vi "ScanParams.vi"(0 "Probe":T2(ring)=enum."Hit U533 Ang6 Sag", 1 "Multiframes?":bool, 7 "hide ftp option? in":bool=TRUE, 9 "location in":u16(ring)=3 items=["VMMC", "U_HI", "Sloan Kett", "Columbia", "RRI Test"], 11 "GaGe Mem":dbl=3.0) -> (4 "Machine Params":T1 {"Scan Info"."sector scan angle" format="%.2f"; "Scan Info"."pivot distance" format="%.2f"; "Scan Info"."delay" format="%.2f"}, 6 "Distance between\nscan lines (um)":sgl, 8 "directory to save data out":path, 10 "hide ftp option? out":bool, 13 "FTP params":T3, 15 "location out":u16(ring)=3 items=["VMMC", "U_HI", "Sloan Kett", "Columbia", "RRI Test"])   [LabVIEW 2022 SP3]
uses:
  MachineParams.ctl
panel:
  out "trig depth pts":dbl
  in  "directory to save data in":path=path "D:/"
  # "Have to set ConterConfig.vi triggers for each machine type."
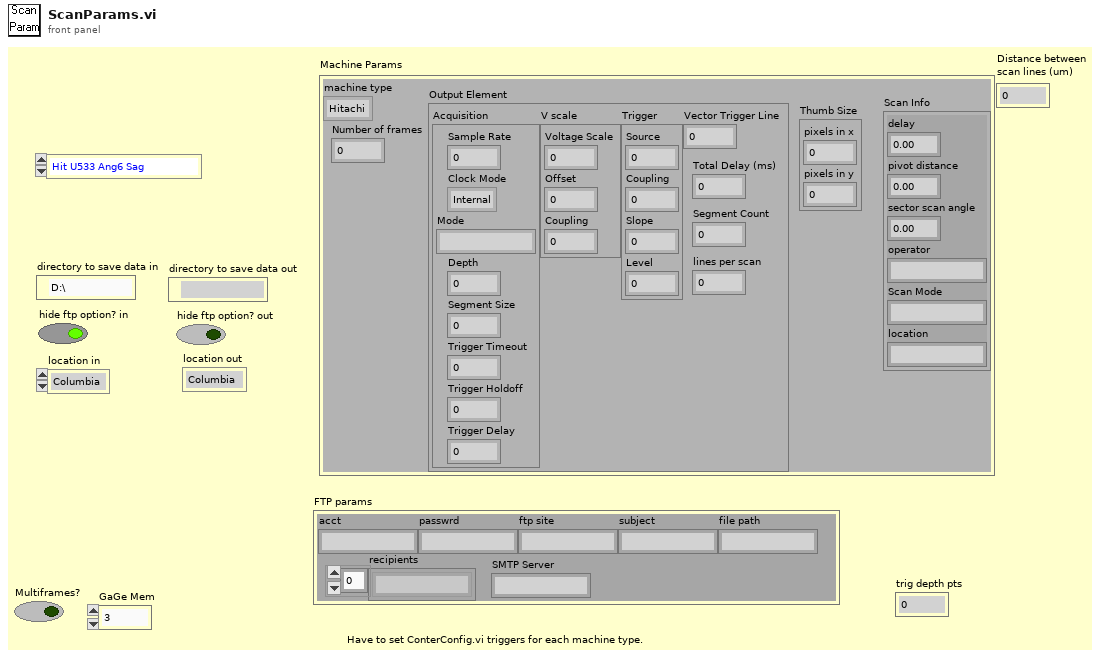
[diagram p1: front panel]
types:
  T1 = typedef "MachineParams.ctl" = cluster{"machine type":enum16{"Hitachi", "B&K 3535", "B&K Hawk"}, "Number of frames":dbl, "Output Element":cluster{"Acquisition":cluster{"Sample Rate":dbl, "Clock Mode":enum16{"Internal", "External", "Reference"}, "Mode":string, "Depth":dbl, "Segment Size":dbl, "Trigger Timeout":dbl, "Trigger Holdoff":dbl, "Trigger Delay":dbl}, "V scale":cluster{"Voltage Scale":i16, "Offset":dbl, "Coupling":u16}, "Trigger":cluster{"Source":u16, "Coupling":u16, "Slope":u16, "Level":dbl}, "Vector Trigger Line":i16, "Total Delay (ms)":dbl, "Segment Count":u32, "lines per scan":i32}, "Thumb Size":cluster{"pixels in x":i16, "pixels in y":i16}, "Scan Info":cluster{"delay":sgl, "pivot distance":sgl, "sector scan angle":sgl, "operator":string, "Scan Mode":string, "location":string}}
  T2 = enum16{"Hitachi-fast (Vx3W)", "Hitachi-detailed (Vx3W)", "Hit U533 Ang5 Trans", "Hit U533 Ang4 Trans", "Hit U533 Ang3 Trans", "Hit U533 Ang6 Sag", "B&K 3535 with TGC", "B&K 3535 with no TGC", "B&K Hawk 8808 (S)", "B&K Hawk 8808 (T)", "B&K Hawk 8808 (Split)", "B&K Hawk 8658 (S)", "B&K Hawk 8658 (T)", "B&K Hawk 8663"}
  T3 = cluster{"acct":string, "passwrd":string, "ftp site":string, "subject":string, "file path":string, "recipients":string[], "SMTP Server":string}
  T4 = cluster{"Acquisition":cluster{"Sample Rate":dbl, "Clock Mode":enum16{"Internal", "External", "Reference"}, "Mode":string, "Depth":dbl, "Segment Size":dbl, "Trigger Timeout":dbl, "Trigger Holdoff":dbl, "Trigger Delay":dbl}, "V scale":cluster{"Voltage Scale":i16, "Offset":dbl, "Coupling":u16}, "Trigger":cluster{"Source":u16, "Coupling":u16, "Slope":u16, "Level":dbl}, "Vector Trigger Line":i16, "Total Delay (ms)":dbl, "Segment Count":u32, "lines per scan":i32}
  T5 = cluster{"delay":sgl, "pivot distance":sgl, "sector scan angle":sgl, "operator":string, "Scan Mode":string, "location":string}
  T6 = cluster{string, string, string, string, string, "recipients":string[], string}
  T7 = cluster{enum16{"Hitachi", "B&K 3535", "B&K Hawk"}, dbl, "Output Element":cluster{"Acquisition":cluster{"Sample Rate":dbl, "Clock Mode":enum16{"Internal", "External", "Reference"}, "Mode":string, "Depth":dbl, "Segment Size":dbl, "Trigger Timeout":dbl, "Trigger Holdoff":dbl, "Trigger Delay":dbl}, "V scale":cluster{"Voltage Scale":i16, "Offset":dbl, "Coupling":u16}, "Trigger":cluster{"Source":u16, "Coupling":u16, "Slope":u16, "Level":dbl}, "Vector Trigger Line":i16, "Total Delay (ms)":dbl, "Segment Count":u32, "lines per scan":i32}, "Thumb Size":cluster{"pixels in x":i16, "pixels in y":i16}, "Scan Info":cluster{"delay":sgl, "pivot distance":sgl, "sector scan angle":sgl, "operator":string, "Scan Mode":string, "location":string}}
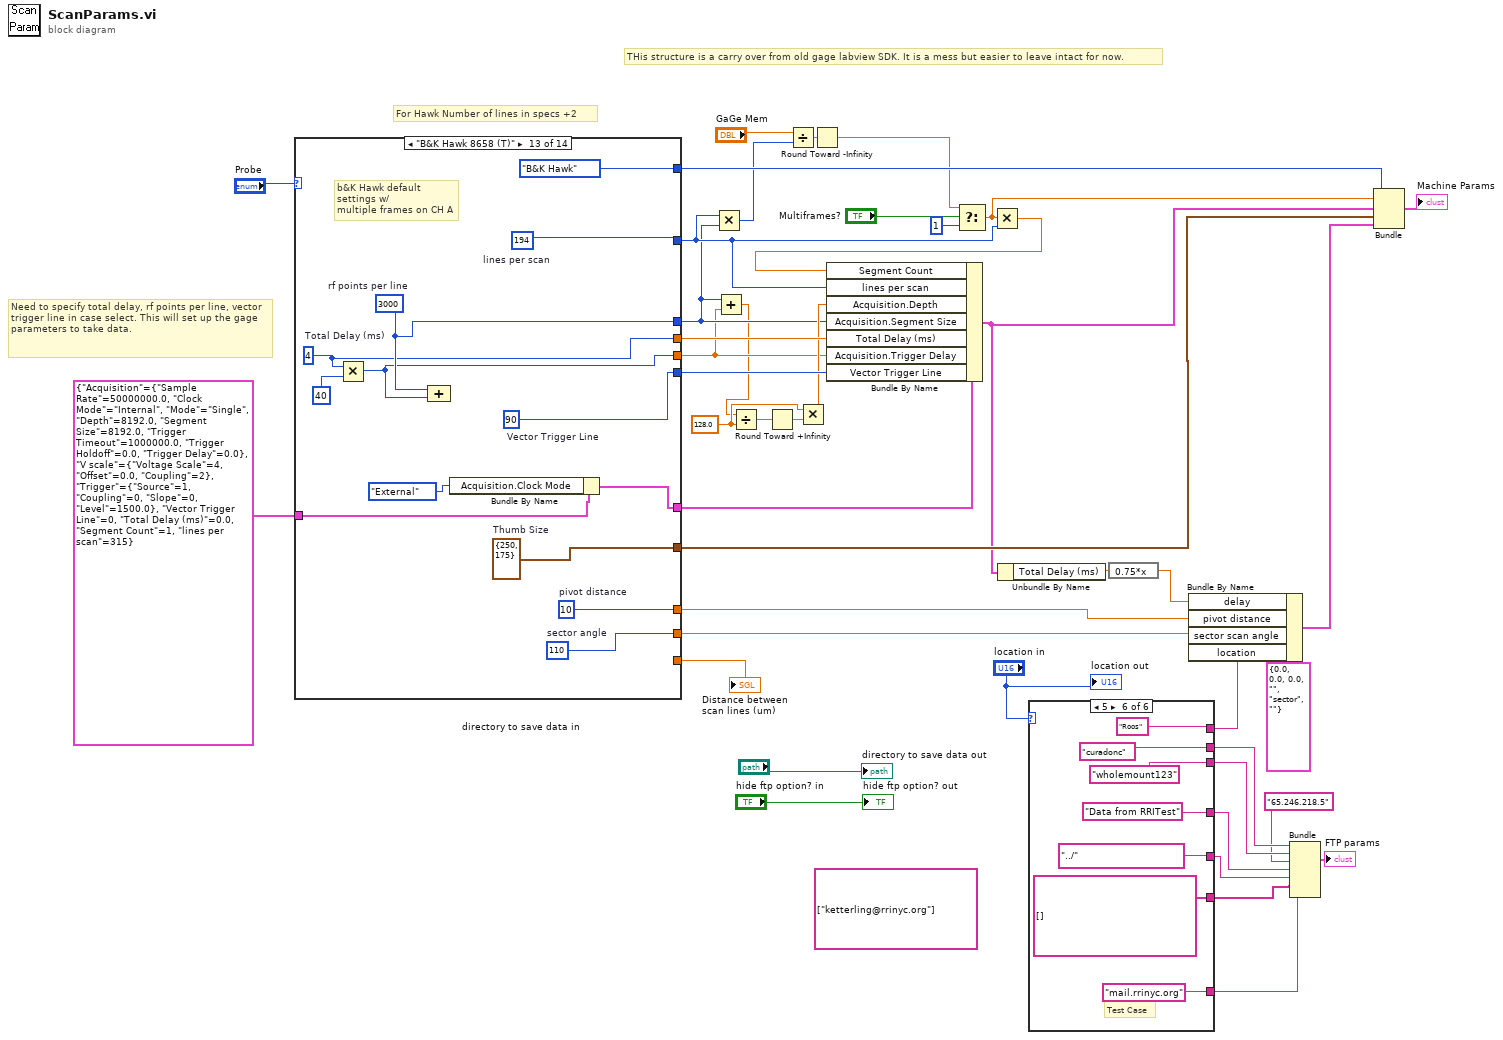
[diagram p0: block diagram]
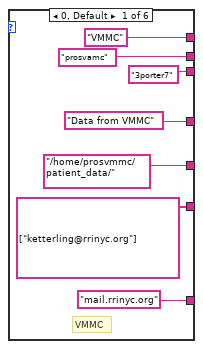
[diagram p2: hidden frame]
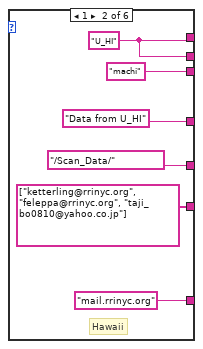
[diagram p3: hidden frame]
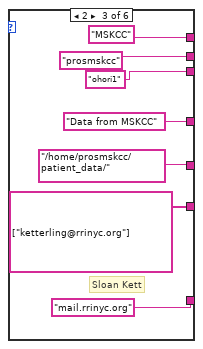
[diagram p4: hidden frame]
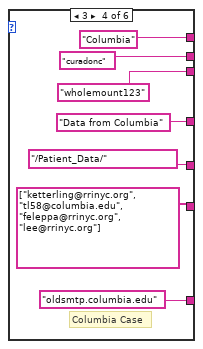
[diagram p5: hidden frame]
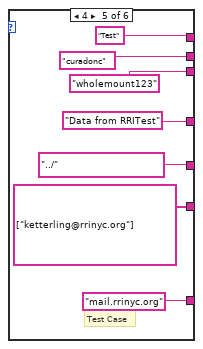
[diagram p6: hidden frame]
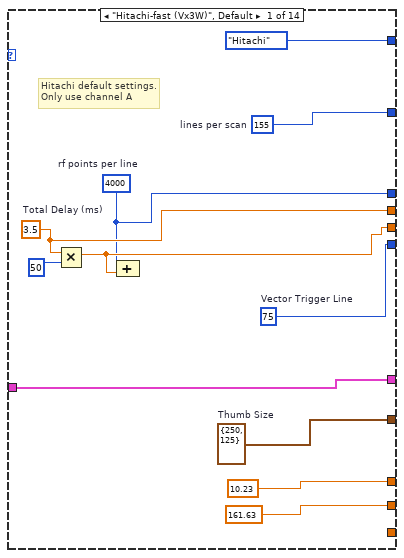
[diagram p7: hidden frame]
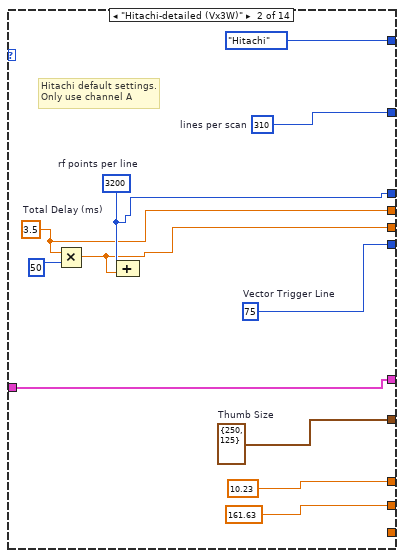
[diagram p8: hidden frame]
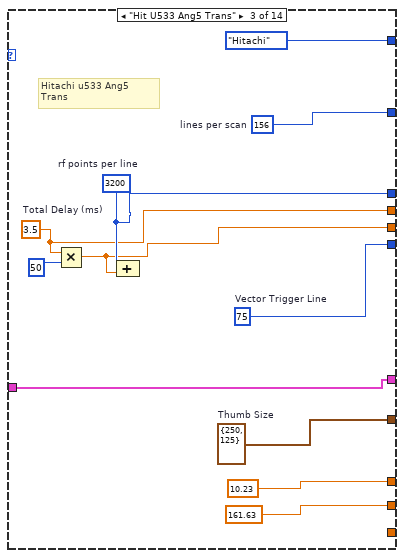
[diagram p9: hidden frame]
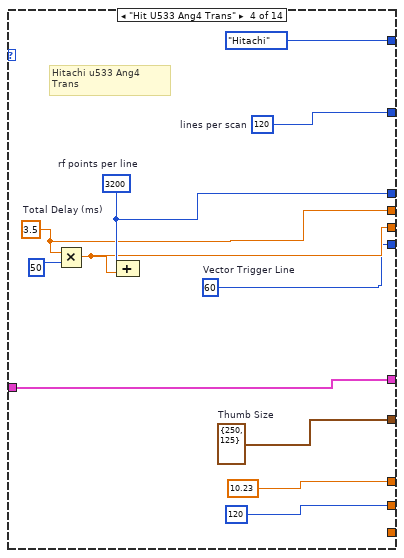
[diagram p10: hidden frame]
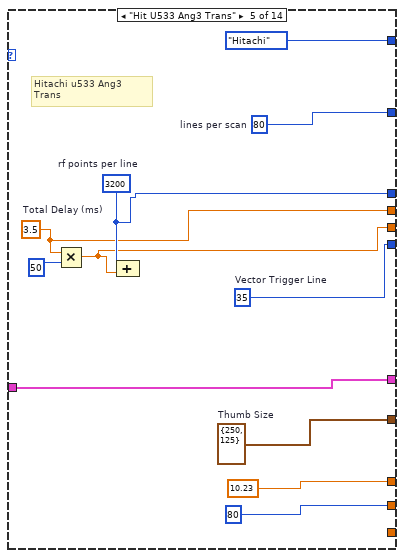
[diagram p11: hidden frame]
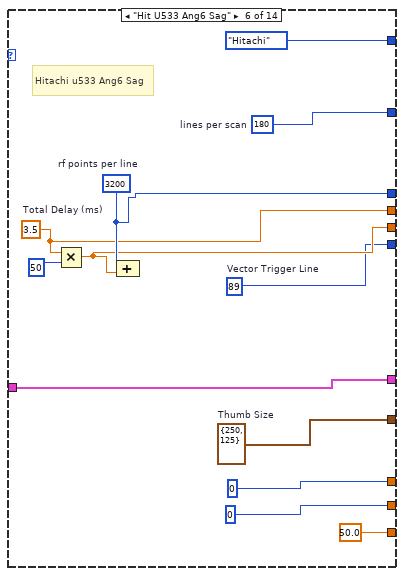
[diagram p12: hidden frame]
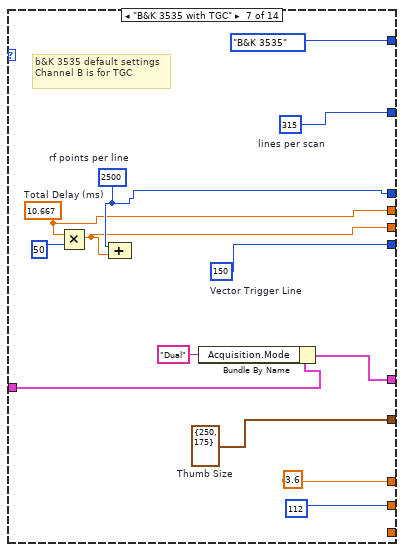
[diagram p13: hidden frame]
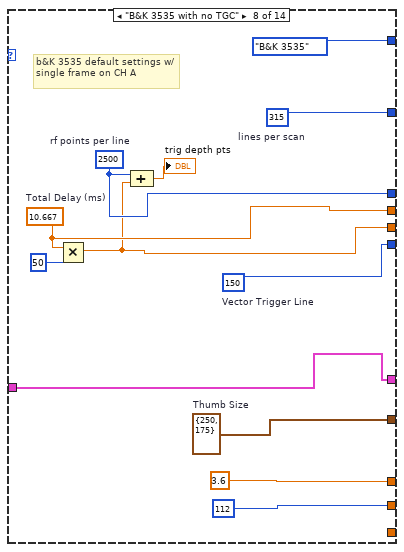
[diagram p14: hidden frame]
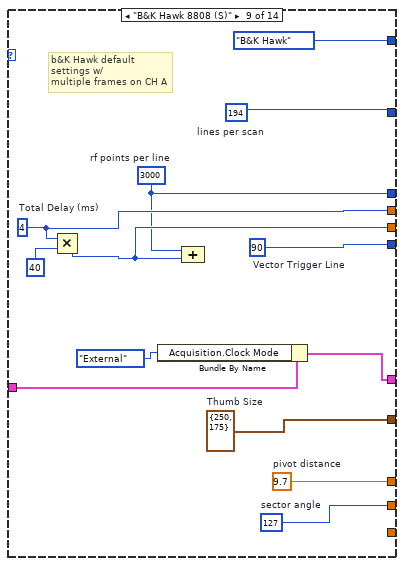
[diagram p15: hidden frame]
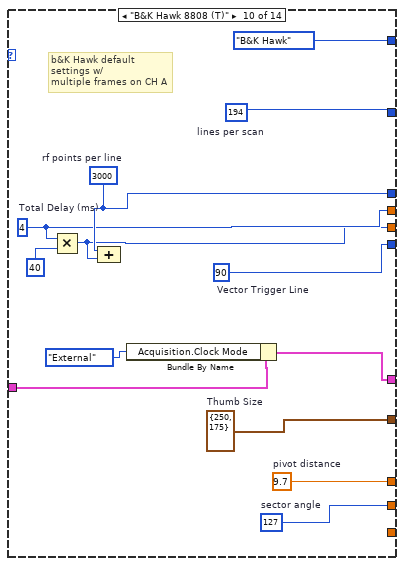
[diagram p16: hidden frame]
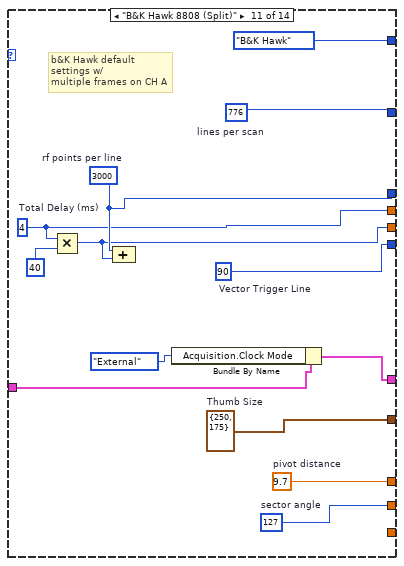
[diagram p17: hidden frame]
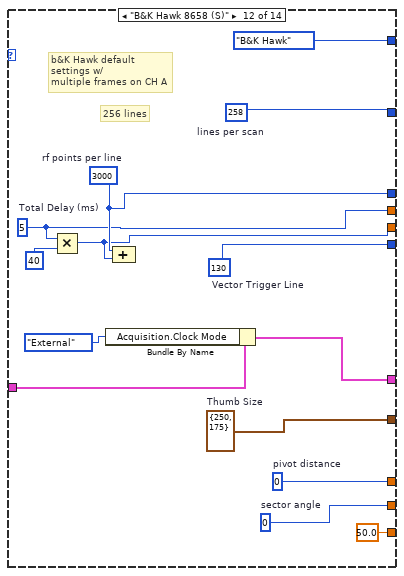
[diagram p18: hidden frame]
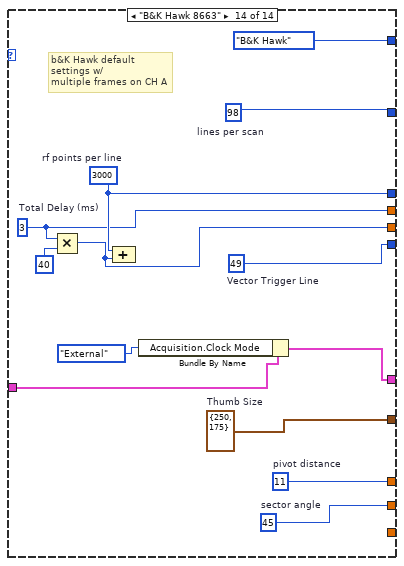
[diagram p19: hidden frame]
diagram:
  w8 = 128.0 ("y")
  (unwired) string[] ["ketterling@rrinyc.org"] ("recipients")
  # "THis structure is a carry over from old gage labview SDK. It is a mess but easier to leave intact for now."
  # "For Hawk Number of lines in specs +2"
  # "Need to specify total delay, rf points per line, vector trigger line in case select. This will set up the gage parameters to take data."
  n1 = case shown="\"B&K Hawk 8658 (T)\"" "Probe" {
    tunnel: [w50 w61 w72 w83 w94 w106 w119 w131 w144 w158 w171 w185 w198 w211] -> w14
    tunnel: [w55 w66 w77 w88 w99 w111 w124 w136 w149 w162 w175 w189 w202 w215] -> w20
    tunnel: [10.23 10.23 10.23 10.23 10.23 0 3.6 3.6 w148 w161 w174 w188 w201 w214] -> w41
    tunnel: [161.63 161.63 161.63 120 80 0 112 112 w147 w160 w173 w187 w200 w213] -> w40
    tunnel: T4 {"Acquisition"={"Sample Rate"=50000000.0, "Clock Mode"=enum."Internal", "Mode"="Single", "Depth"=8192.0, "Segment Size"=8192.0, "Trigger Timeout"=1000000.0, "Trigger Holdoff"=0.0, "Trigger Delay"=0.0}, "V scale"={"Voltage Scale"=4, "Offset"=0.0, "Coupling"=2}, "Trigger"={"Source"=1, "Coupling"=0, "Slope"=0, "Level"=1500.0}, "Vector Trigger Line"=0, "Total Delay (ms)"=0.0, "Segment Count"=1, "lines per scan"=315} ("Output Element") -> [w48 w56 w68 w78 w89 w101 w113 w125 w140 w154 w168 w182 w195 w207]
    tunnel: [enum16{"Hitachi", "B&K 3535", "B&K Hawk"}."Hitachi" enum16{"Hitachi", "B&K 3535", "B&K Hawk"}."Hitachi" enum16{"Hitachi", "B&K 3535", "B&K Hawk"}."Hitachi" enum16{"Hitachi", "B&K 3535", "B&K Hawk"}."Hitachi" enum16{"Hitachi", "B&K 3535", "B&K Hawk"}."Hitachi" enum16{"Hitachi", "B&K 3535", "B&K Hawk"}."Hitachi" enum16{"Hitachi", "B&K 3535", "B&K Hawk"}."B&K 3535" enum16{"Hitachi", "B&K 3535", "B&K Hawk"}."B&K 3535" enum16{"Hitachi", "B&K 3535", "B&K Hawk"}."B&K Hawk" enum16{"Hitachi", "B&K 3535", "B&K Hawk"}."B&K Hawk" enum16{"Hitachi", "B&K 3535", "B&K Hawk"}."B&K Hawk" enum16{"Hitachi", "B&K 3535", "B&K Hawk"}."B&K Hawk" enum16{"Hitachi", "B&K 3535", "B&K Hawk"}."B&K Hawk" enum16{"Hitachi", "B&K 3535", "B&K Hawk"}."B&K Hawk"] -> w38
    tunnel: [w45 w60 w71 w82 w93 w105 w118 w129 w137 w152 w165 w180 w192 w205] -> w6
    tunnel: [w47 w58 w67 w80 w91 w103 w116 w127 w142 w150 w163 w178 w190 w203] -> w5
    tunnel: [w46 w59 w70 w81 w92 w104 w117 w128 w143 w151 w164 w179 w191 w204] -> w18
    tunnel: [w49 w57 w69 w79 w90 w102 w115 w126 w141 w153 w166 w181 w193 w209] -> w17
    tunnel: [w48 w56 w68 w78 w89 w101 w114 w125 w138 w155 w167 w176 w194 w206] -> w16
    tunnel: [_ _ _ _ _ sgl 50.0 ("Distance between\nscan lines (mm)") _ _ _ _ _ sgl 50.0 ("Distance between\nscan lines (mm)") _ _] -> w11
    frame "Hitachi-fast (Vx3W)", Default {
      w55 = cluster{"pixels in x":i16, "pixels in y":i16} {"pixels in x"=250, "pixels in y"=125}  # Thumb Size
      w49 = i16 75  # Vector Trigger Line
      w46 = 3.5  # Total Delay (ms)
      w50 = 155  # lines per scan
      w45 = 4000  # rf points per line
      # "Hitachi default settings.\nOnly use channel A"
      n2 = Multiply(x=w46, y=50) -> (x*y=w47:dbl)
      n3 = Compound Arithmetic op=unknown(w45, w47) -> ()  [unwired: 1 out]
    }
    frame "Hitachi-detailed (Vx3W)" {
      w66 = cluster{"pixels in x":i16, "pixels in y":i16} {"pixels in x"=250, "pixels in y"=125}  # Thumb Size
      w57 = i16 75  # Vector Trigger Line
      w59 = 3.5  # Total Delay (ms)
      w61 = 310  # lines per scan
      w60 = 3200  # rf points per line
      # "Hitachi default settings.\nOnly use channel A"
      n4 = Multiply(x=w59, y=50) -> (x*y=w58:dbl)
      n5 = Compound Arithmetic op=unknown(w60, w58) -> ()  [unwired: 1 out]
    }
    frame "Hit U533 Ang5 Trans" {
      w77 = cluster{"pixels in x":i16, "pixels in y":i16} {"pixels in x"=250, "pixels in y"=125}  # Thumb Size
      w69 = i16 75  # Vector Trigger Line
      w70 = 3.5  # Total Delay (ms)
      w72 = 156  # lines per scan
      w71 = 3200  # rf points per line
      # "Hitachi u533 Ang5 Trans"
      n6 = Multiply(x=w70, y=50) -> (x*y=w67:dbl)
      n7 = Compound Arithmetic op=unknown(w71, w67) -> ()  [unwired: 1 out]
    }
    frame "Hit U533 Ang4 Trans" {
      w88 = cluster{"pixels in x":i16, "pixels in y":i16} {"pixels in x"=250, "pixels in y"=125}  # Thumb Size
      w79 = i16 60  # Vector Trigger Line
      w81 = 3.5  # Total Delay (ms)
      w83 = 120  # lines per scan
      w82 = 3200  # rf points per line
      # "Hitachi u533 Ang4 Trans"
      n8 = Multiply(x=w81, y=50) -> (x*y=w80:dbl)
      n9 = Compound Arithmetic op=unknown(w82, w80) -> ()  [unwired: 1 out]
    }
    frame "Hit U533 Ang3 Trans" {
      w99 = cluster{"pixels in x":i16, "pixels in y":i16} {"pixels in x"=250, "pixels in y"=125}  # Thumb Size
      w90 = i16 35  # Vector Trigger Line
      w92 = 3.5  # Total Delay (ms)
      w94 = 80  # lines per scan
      w93 = 3200  # rf points per line
      # "Hitachi u533 Ang3 Trans"
      n10 = Multiply(x=w92, y=50) -> (x*y=w91:dbl)
      n11 = Compound Arithmetic op=unknown(w93, w91) -> ()  [unwired: 1 out]
    }
    frame "Hit U533 Ang6 Sag" {
      w111 = cluster{"pixels in x":i16, "pixels in y":i16} {"pixels in x"=250, "pixels in y"=125}  # Thumb Size
      w102 = i16 89  # Vector Trigger Line
      w104 = 3.5  # Total Delay (ms)
      w106 = 180  # lines per scan
      w105 = 3200  # rf points per line
      # "Hitachi u533 Ang6 Sag"
      n12 = Multiply(x=w104, y=50) -> (x*y=w103:dbl)
      n13 = Compound Arithmetic op=unknown(w105, w103) -> ()  [unwired: 1 out]
    }
    frame "B&K 3535 with TGC" {
      w117 = 10.667  # Total Delay (ms)
      w124 = cluster{"pixels in x":i16, "pixels in y":i16} {"pixels in x"=250, "pixels in y"=175}  # Thumb Size
      w115 = i16 150  # Vector Trigger Line
      w119 = 315  # lines per scan
      w118 = 2500  # rf points per line
      # "b&K 3535 default settings Channel B is for TGC"
      n14 = Multiply(x=w117, y=50) -> (x*y=w116:dbl)
      n15 = Compound Arithmetic op=unknown(w118, w116) -> ()  [unwired: 1 out]
      n16 = Bundle By Name(cluster=w113, "Acquisition.Mode"="Dual") -> (w114:T4)
    }
    frame "B&K 3535 with no TGC" {
      w136 = cluster{"pixels in x":i16, "pixels in y":i16} {"pixels in x"=250, "pixels in y"=175}  # Thumb Size
      w126 = i16 150  # Vector Trigger Line
      w128 = 10.667  # Total Delay (ms)
      w131 = 315  # lines per scan
      w129 = 2500  # rf points per line
      # "b&K 3535 default settings w/\nsingle frame on CH A"
      n17 = Multiply(x=w128, y=50) -> (x*y=w127:dbl)
      n18 = Compound Arithmetic op=unknown(w129, w127) -> (→"trig depth pts":dbl)
    }
    frame "B&K Hawk 8808 (S)" {
      w149 = cluster{"pixels in x":i16, "pixels in y":i16} {"pixels in x"=250, "pixels in y"=175}  # Thumb Size
      w141 = i16 90  # Vector Trigger Line
      w143 = 4  # Total Delay (ms)
      w147 = 127  # sector angle
      w148 = 9.7  # pivot distance
      w144 = 194  # lines per scan
      w137 = 3000  # rf points per line
      # "b&K Hawk default settings w/\nmultiple frames on CH A"
      n19 = Multiply(x=w143, y=40) -> (x*y=w142:i32)
      n20 = Bundle By Name(cluster=w140, "Acquisition.Clock Mode"=enum16{"Internal", "External", "Reference"}."External" ("Clock Mode")) -> (w138:T4)
      n21 = Compound Arithmetic op=unknown(w137, w142) -> ()  [unwired: 1 out]
    }
    frame "B&K Hawk 8808 (T)" {
      w162 = cluster{"pixels in x":i16, "pixels in y":i16} {"pixels in x"=250, "pixels in y"=175}  # Thumb Size
      w153 = i16 90  # Vector Trigger Line
      w151 = 4  # Total Delay (ms)
      w160 = 127  # sector angle
      w161 = 9.7  # pivot distance
      w158 = 194  # lines per scan
      w152 = 3000  # rf points per line
      # "b&K Hawk default settings w/\nmultiple frames on CH A"
      n22 = Multiply(x=w151, y=40) -> (x*y=w150:i32)
      n23 = Compound Arithmetic op=unknown(w152, w150) -> ()  [unwired: 1 out]
      n24 = Bundle By Name(cluster=w154, "Acquisition.Clock Mode"=enum16{"Internal", "External", "Reference"}."External" ("Clock Mode")) -> (w155:T4)
    }
    frame "B&K Hawk 8808 (Split)" {
      w175 = cluster{"pixels in x":i16, "pixels in y":i16} {"pixels in x"=250, "pixels in y"=175}  # Thumb Size
      w166 = i16 90  # Vector Trigger Line
      w164 = 4  # Total Delay (ms)
      w173 = 127  # sector angle
      w174 = 9.7  # pivot distance
      w171 = 776  # lines per scan
      w165 = 3000  # rf points per line
      # "b&K Hawk default settings w/\nmultiple frames on CH A"
      n25 = Multiply(x=w164, y=40) -> (x*y=w163:i32)
      n26 = Compound Arithmetic op=unknown(w165, w163) -> ()  [unwired: 1 out]
      n27 = Bundle By Name(cluster=w168, "Acquisition.Clock Mode"=enum16{"Internal", "External", "Reference"}."External" ("Clock Mode")) -> (w167:T4)
    }
    frame "B&K Hawk 8658 (S)" {
      w189 = cluster{"pixels in x":i16, "pixels in y":i16} {"pixels in x"=250, "pixels in y"=175}  # Thumb Size
      w181 = i16 130  # Vector Trigger Line
      w179 = 5  # Total Delay (ms)
      w187 = 0  # sector angle
      w188 = 0  # pivot distance
      w185 = 258  # lines per scan
      w180 = 3000  # rf points per line
      # "256 lines"
      # "b&K Hawk default settings w/\nmultiple frames on CH A"
      n28 = Multiply(x=w179, y=40) -> (x*y=w178:i32)
      n29 = Bundle By Name(cluster=w182, "Acquisition.Clock Mode"=enum16{"Internal", "External", "Reference"}."External" ("Clock Mode")) -> (w176:T4)
      n30 = Compound Arithmetic op=unknown(w180, w178) -> ()  [unwired: 1 out]
    }
    frame "B&K Hawk 8658 (T)" {
      w202 = cluster{"pixels in x":i16, "pixels in y":i16} {"pixels in x"=250, "pixels in y"=175}  # Thumb Size
      w193 = i16 90  # Vector Trigger Line
      w191 = 4  # Total Delay (ms)
      w200 = 110  # sector angle
      w201 = 10  # pivot distance
      w198 = 194  # lines per scan
      w192 = 3000  # rf points per line
      # "b&K Hawk default settings w/\nmultiple frames on CH A"
      n31 = Multiply(x=w191, y=40) -> (x*y=w190:i32)
      n32 = Compound Arithmetic op=unknown(w192, w190) -> ()  [unwired: 1 out]
      n33 = Bundle By Name(cluster=w195, "Acquisition.Clock Mode"=enum16{"Internal", "External", "Reference"}."External" ("Clock Mode")) -> (w194:T4)
    }
    frame "B&K Hawk 8663" {
      w215 = cluster{"pixels in x":i16, "pixels in y":i16} {"pixels in x"=250, "pixels in y"=175}  # Thumb Size
      w209 = i16 49  # Vector Trigger Line
      w204 = 3  # Total Delay (ms)
      w213 = 45  # sector angle
      w214 = 11  # pivot distance
      w211 = 98  # lines per scan
      w205 = 3000  # rf points per line
      # "b&K Hawk default settings w/\nmultiple frames on CH A"
      n34 = Multiply(x=w204, y=40) -> (x*y=w203:i32)
      n35 = Compound Arithmetic op=unknown(w205, w203) -> ()  [unwired: 1 out]
      n36 = Bundle By Name(cluster=w207, "Acquisition.Clock Mode"=enum16{"Internal", "External", "Reference"}."External" ("Clock Mode")) -> (w206:T4)
    }
  }
  "Distance between\nscan lines (um)" <- w11
  n37 = Multiply(x=w14, y=w6) -> (x*y=w27:i32)
  n38 = Add(x=w6, y=w5) -> (x+y=w4:dbl)
  n39 = Divide(x=w4, y=w8) -> (x/y=w10:dbl)
  n40 = Round Toward +Infinity(x=w10) -> (ceil(x): smallest int >= x=w9:dbl)
  n41 = Divide(x="GaGe Mem", y=w27) -> (x/y=w28:dbl)
  n42 = Multiply(x=w8, y=w9) -> (x*y=w7:dbl)
  n43 = Round Toward -Infinity(1:w28) -> (0:w24:dbl)
  n44 = Select(t=w24, s="Multiframes?", f=1) -> (s? t:f=w23:dbl)
  n45 = Multiply(x=w23, y=w14) -> (x*y=w15:dbl)
  n46 = Bundle By Name(cluster=w16, "Segment Count"=w15, "lines per scan"=w14, "Acquisition.Depth"=w7, "Acquisition.Segment Size"=w6, "Total Delay (ms)"=w18, "Acquisition.Trigger Delay"=w5, "Vector Trigger Line"=w17) -> (w13:T4)
  n47 = Unbundle By Name(w13) -> ("Total Delay (ms)"=w3:dbl)
  n48 = case shown="5" "location in" {
    tunnel: ["/home/prosvmmc/patient_data/" "/Scan_Data/" "/home/prosmskcc/patient_data/" "/Patient_Data/" "../" "../"] -> w33
    tunnel: ["prosvamc" w224 "prosmskcc" "curadonc" "curadonc" "curadonc"] -> w36
    tunnel: ["3porter7" "machi" "ohori1" "wholemount123" "wholemount123" "wholemount123"] -> w35
    tunnel: ["Data from VMMC" "Data from U_HI" "Data from MSKCC" "Data from Columbia" "Data from RRITest" "Data from RRITest"] -> w34
    tunnel: ["VMMC" w224 "MSKCC" "Columbia" "Test" "Roos"] -> w32
    tunnel: ["mail.rrinyc.org" "mail.rrinyc.org" "mail.rrinyc.org" "oldsmtp.columbia.edu" "mail.rrinyc.org" "mail.rrinyc.org"] -> w29
    tunnel: [string[] ["ketterling@rrinyc.org"] ("recipients") string[] ["ketterling@rrinyc.org", "feleppa@rrinyc.org", "taji_bo0810@yahoo.co.jp"] ("recipients") string[] ["ketterling@rrinyc.org"] ("recipients") string[] ["ketterling@rrinyc.org", "tl58@columbia.edu", "feleppa@rrinyc.org", "lee@rrinyc.org"] ("recipients") string[] ["ketterling@rrinyc.org"] ("recipients") string[] [] ("recipients")] -> w22
    frame 0, Default {
      # "VMMC"
    }
    frame 1 {
      w224 = "U_HI"
      # "Hawaii"
    }
    frame 2 {
      # "Sloan Kett"
    }
    frame 3 {
      # "Columbia Case"
    }
    frame 4 {
      # "Test Case"
    }
    frame 5 {
      # "Test Case"
    }
  }
  n49 = expression code="0.75*x"(w3) -> (w2:dbl)
  n50 = Bundle By Name(cluster=T5 {"delay"=0.0, "pivot distance"=0.0, "sector scan angle"=0.0, "operator"="", "Scan Mode"="sector", "location"=""} ("Scan Info"), "delay"=w2, "pivot distance"=w41, "sector scan angle"=w40, "location"=w32) -> (w1:T5)
  n51 = Bundle(w36, w35, "65.246.218.5", w34, w33, "recipients"=w22, w29) -> (→"FTP params":T6)  [unwired: 1 out]
  n52 = Bundle(w38, w23, "Output Element"=w13, "Thumb Size"=w20, "Scan Info"=w1) -> (→"Machine Params":T7)  [unwired: 1 out]
  "directory to save data out" <- "directory to save data in"
  "hide ftp option? out" <- "hide ftp option? in"
  "location out" <- "location in"
